vi "Process.vi"(11 "Actor":refnum<class "Main View.lvclass">) -> ()   [LabVIEW 2021, in "Main View.lvclass"]
uses:
  Main View.lvclass
  Element/Element.lvclass/Element.ctl
  Motion/Motion.lvclass/Motion.ctl
  Vector 2D/Vector 2D.lvclass/Vector 2D.ctl
  Re-use Libraries/Minimal Actor Framework/Actors/Base Actor/Actor/Front Panel State.ctl
  Re-use Libraries/Minimal Actor Framework/Actors/Base Actor/Actor/Actor.lvclass
  Re-use Libraries/Minimal Actor Framework/Messaging/Message/Message.lvclass
  Actors/Error Handler/API/Error Handler Actor API.lvclass
  Re-use Libraries/Utility/Utility.lvlib
  Actors/Main Controller/API/Main Controller Actor API.lvclass
  Actors/Main Controller/Actor/Player.ctl
  Actors/Main Controller/Actor/Main Controller Actor.lvclass
  Globals.vi
  Element/Element.lvclass
  Motion/Motion.lvclass
  Vector 2D/Vector 2D.lvclass
  Actors/Main Controller/Actor/Player Icon.ctl
panel:
  in  "Player 2 Position":cluster{"X":i32, "Y":i32}={"X"=2000, "Y"=2000} {"Y" scale=0.0..6400.0; "X" scale=0.0..8192.0}
  in  "Player 1 Position":cluster{"X":i32, "Y":i32}={"X"=1000, "Y"=1000} {"Y" scale=0.0..6400.0; "X" scale=0.0..8192.0}
  in  "Player 2":T1=1
  in  "Player 1":T1
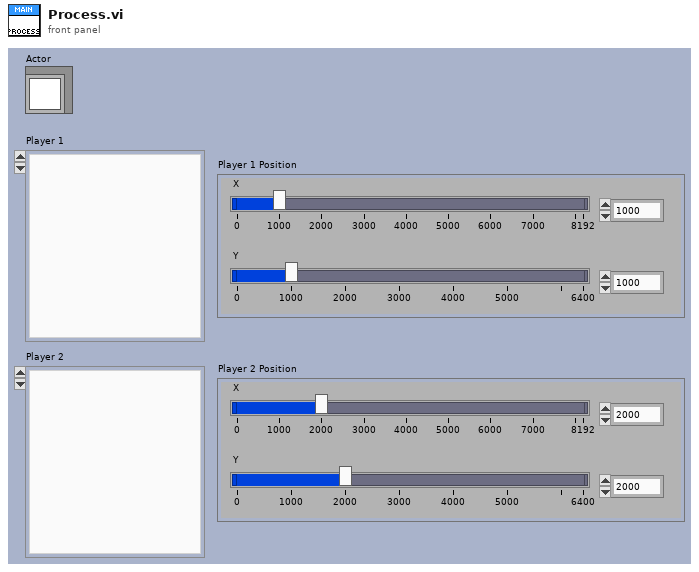
[diagram p1: front panel]
types:
  T1 = typedef "Main Controller Actor.lvclass/Player Icon.ctl" = u16
  T2 = typedef "Actor.lvclass/Front Panel State.ctl" = enum32{"Invalid", "Standard", "Closed", "Hidden", "Minimized", "Maximized"}
  T3 = typedef "Main Controller Actor.lvclass/Player.ctl" = enum16{"1", "2"}
  T4 = cluster{"Actor":refnum<event-registration>, "Main Controller":refnum<event-registration>}
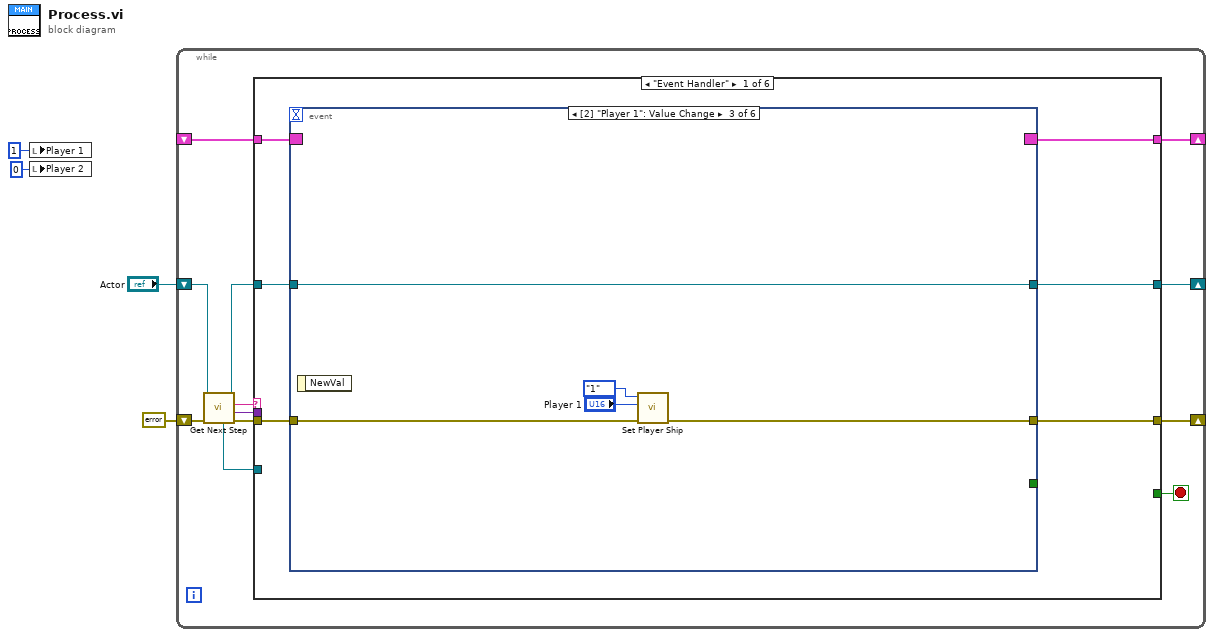
[diagram p0: block diagram]
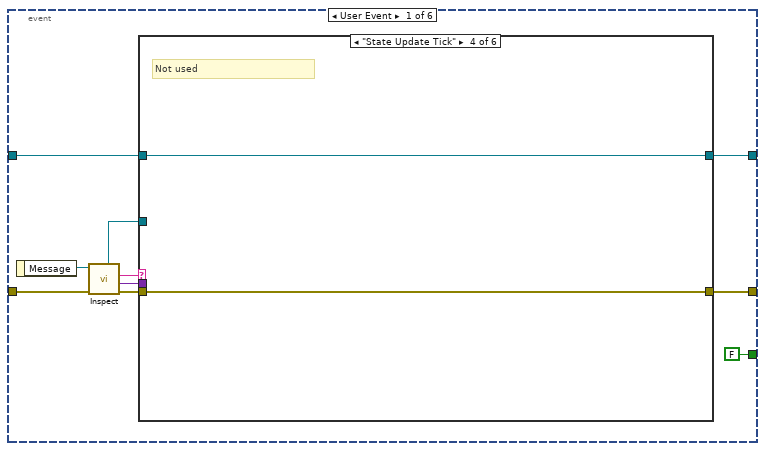
[diagram p2: hidden frame]
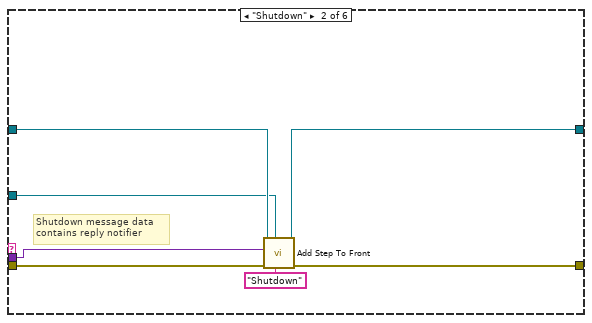
[diagram p4: hidden frame]
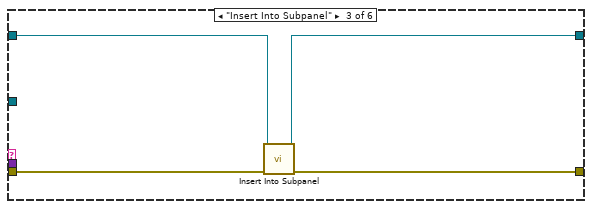
[diagram p5: hidden frame]
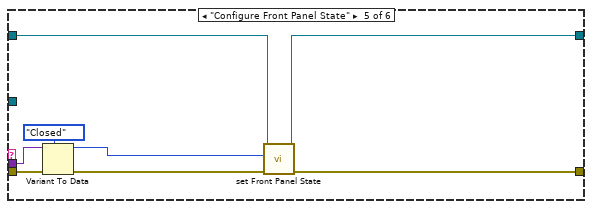
[diagram p6: hidden frame]
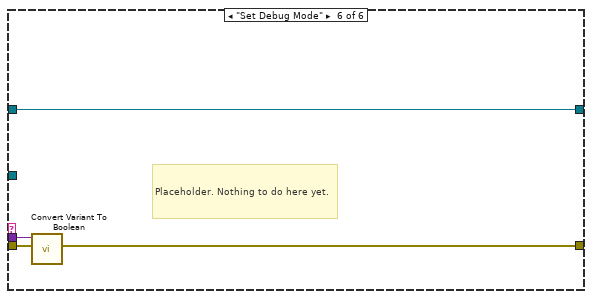
[diagram p7: hidden frame]
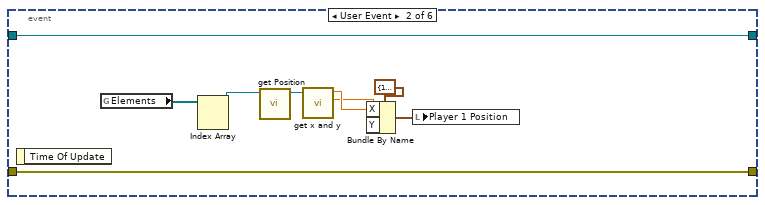
[diagram p8: hidden frame]
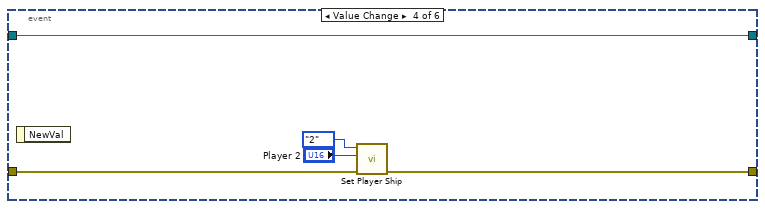
[diagram p9: hidden frame]
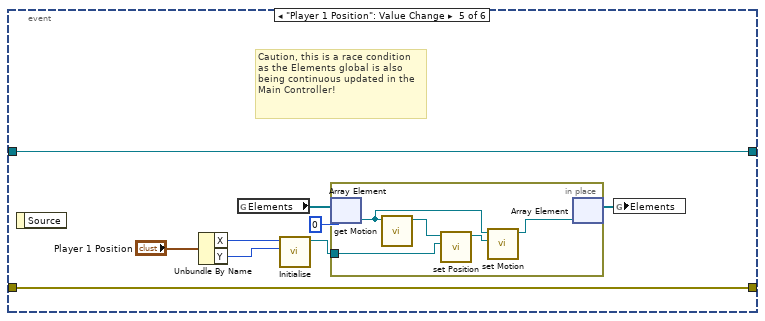
[diagram p10: hidden frame]
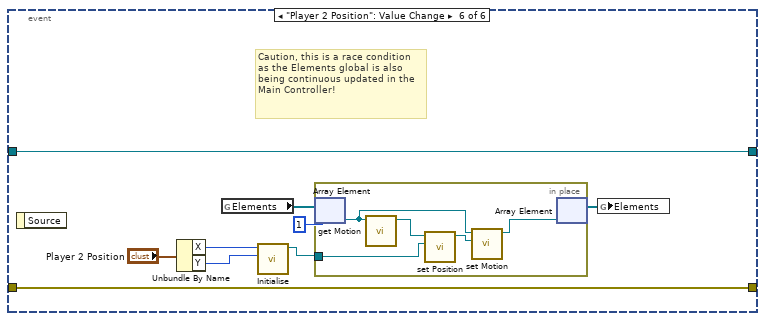
[diagram p11: hidden frame]
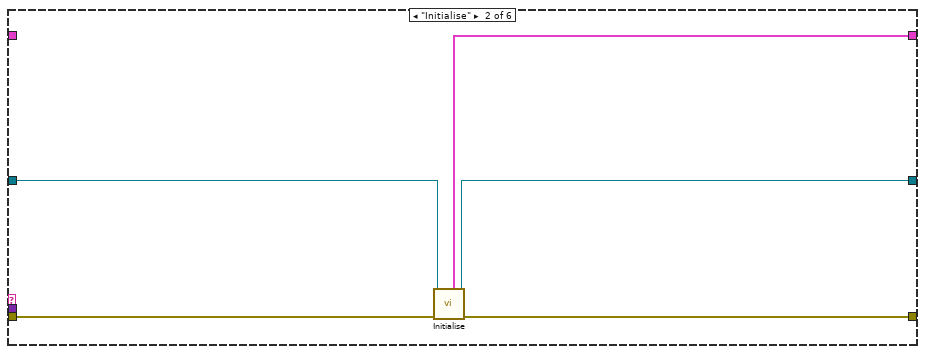
[diagram p12: hidden frame]
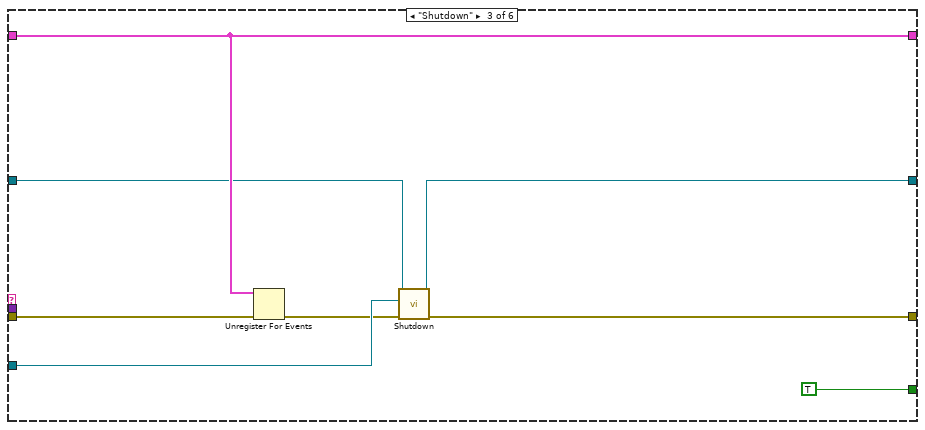
[diagram p13: hidden frame]
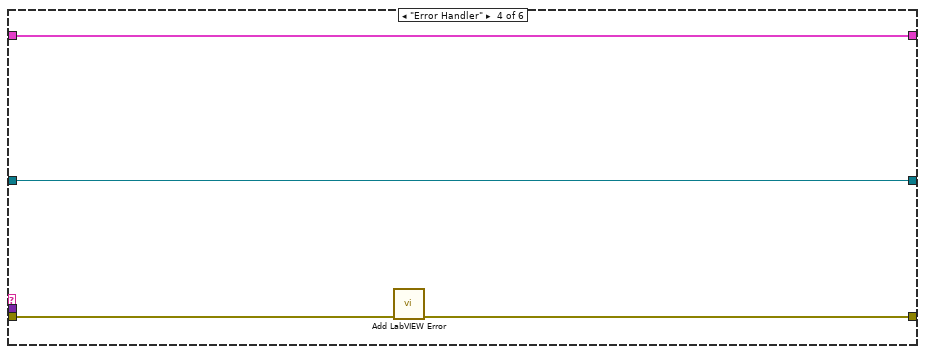
[diagram p14: hidden frame]
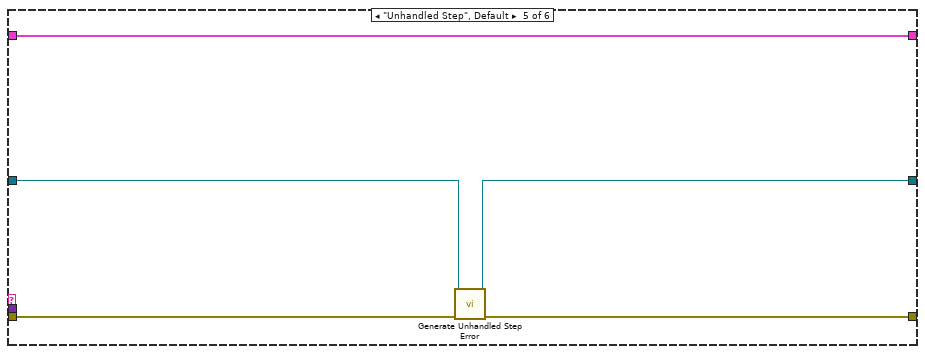
[diagram p15: hidden frame]
diagram:
  n1 = local write "Player 1"(T1 1 ("Player 1")) -> ()
  n2 = local write "Player 2"(T1 0 ("Player 2")) -> ()
  n3 = while {
    shift-right: [w7] -> _
    shift-left: "Actor" -> [w15]
    shift-right: [w12] -> _
    shift-left: _ -> [w11]
    shift-right: [w6] -> _
    shift-left: errorcluster {"status"=FALSE, "code"=0, "source"=""} ("error constant") -> [w9]
    stop <- w16 stop-if-true
    n4 = call-dynamic "Get Next Step.vi"("error in (no error)"=w9, "Actor in"=w15) -> ("error out"=w10:errorcluster, "Parameter"=w13:variant, "Step"=w8:string, "Actor out"=w14:refnum<class "Main View.lvclass">, "Reply Channel"=w5:refnum<notifier>)  [unwired: 5 in]
    n5 = case shown="\"Event Handler\"" w8 {
      tunnel: [_ _ TRUE _ _ _] -> w16
      tunnel: w14 -> [w22 w109 w117 w120 w127 w130]
      tunnel: [w21 w108 w116 w120 w126 w130] -> w7
      tunnel: w13 -> [_ _ _ _ _ _]
      tunnel: [w19 w111 w118 w123 w128 w131] -> w12
      tunnel: w11 -> [w20 _ w118 w123 w128 w131]
      tunnel: w10 -> [w18 w110 w114 w122 w125 w129]
      tunnel: [w17 w107 w112 w121 w124 w129] -> w6
      tunnel: w5 -> [_ _ w115 _ _ _]
      frame "Event Handler" {
        n6 = event shown="[2] \"Player 1\": Value Change" {
          selector: w20 -> [_ _ _ _ _ _]
          dyn-events: [_ _ _ _ _ _] -> w19
          timeout: _ -> [_ _ _ _ _ _]
          tunnel: w22 -> [w32 w68 w73 w78 w83 w101]
          tunnel: [w31 w68 w73 w78 w83 w101] -> w21
          tunnel: w18 -> [w29 w67 w71 w76 w87 w100]
          tunnel: [w30 w67 w70 w75 w87 w100] -> w17
          tunnel: [FALSE _ _ _ _ _] -> _
          event User Event {
            n7 = event-data() -> ("Message"=w28:refnum<class "Message.lvclass">)  [unwired: 1 in]
            n8 = call "Inspect.vi"("error in (no error)"=w29, "Message in"=w28) -> ("error out"=w25:errorcluster, "Data"=w26:variant, "Name"=w27:string, "Reply Channel"=w24:refnum<notifier>)  [unwired: 5 in, 1 out]
            n9 = case shown="\"State Update Tick\"" w27 {
              tunnel: w32 -> [w34 w41 w45 w47 w55 w59]
              tunnel: [w34 w40 w44 w47 w54 w59] -> w31
              tunnel: w25 -> [w33 w38 w43 w46 w51 w57]
              tunnel: [w33 w37 w42 w46 w53 w56] -> w30
              tunnel: w26 -> [_ w36 _ _ w52 w58]
              tunnel: w24 -> [_ w35 _ _ _ _]
              frame Default {
              }
              frame "Shutdown" {
                # "Shutdown message data contains reply notifier"
                n10 = call-dynamic "Add Step To Front.vi"("Step Name"="Shutdown", "Reply Channel"=w35, "error in (no error)"=w38, "Parameter"=w36, "Actor in"=w41) -> ("error out"=w37:errorcluster, "Actor out"=w40:refnum<class "Main View.lvclass">)  [unwired: 5 in]
              }
              frame "Insert Into Subpanel" {
                n11 = call-dynamic "Insert Into Subpanel.vi"("error in (no error)"=w43, "Actor in"=w45) -> ("error out"=w42:errorcluster, "Actor out"=w44:refnum<class "Main View.lvclass">)  [unwired: 8 in]
              }
              frame "State Update Tick" {
                # "Not used"
              }
              frame "Configure Front Panel State" {
                n12 = Variant To Data(error in=w51, type=Front_Panel_State."Closed" ("Front Panel State"), Variant=w52) -> (data=w48:T2, error out=w50:errorcluster)
                n13 = call-dynamic "set Front Panel State.vi"("error in (no error)"=w50, "Front Panel State"=w48, "Actor in"=w55) -> ("error out"=w53:errorcluster, "Actor out"=w54:refnum<class "Main View.lvclass">)  [unwired: 7 in]
              }
              frame "Set Debug Mode" {
                # "Placeholder. Nothing to do here yet."
                n14 = call "Convert Variant To Boolean.vi"("error in (no error)"=w57, "Variant"=w58) -> ("error out"=w56:errorcluster)  [unwired: 8 in, 1 out]
              }
            }
          }
          event User Event {
            n15 = event-data() -> ()  [unwired: 1 in, 1 out]
            n16 = global read "Globals.vi" "Elements"() -> (w66:refnum<class "Element.lvclass">[])
            n17 = Index Array(array=w66) -> (element #1=w65:refnum<class "Element.lvclass">)  [unwired: 2 in, 1 out]
            n18 = call "get Position.vi"("Element in"=w65) -> ("Position"=w64:refnum<class "Vector 2D.lvclass">)  [unwired: 10 in]
            n19 = call "get x and y.vi"("Vector 2D in"=w64) -> ("y"=w61:sgl, "x"=w62:sgl)  [unwired: 9 in]
            n20 = Bundle By Name(cluster=cluster{"X":i32, "Y":i32} {"X"=1000, "Y"=1000} ("Player 1 Position"), "X"=w62, "Y"=w61) -> (w63:cluster{"X":i32, "Y":i32})
            n21 = local write "Player 1 Position"(w63) -> ()
          }
          event Value Change {
            n22 = event-data() -> ()  [unwired: 1 in, 1 out]
            n23 = call "Set Player Ship.vi"("error in (no error)"=w71, "Ship"="Player 1", "Player"=Player."1") -> ("error out"=w70:errorcluster)  [unwired: 8 in]
          }
          event Value Change {
            n24 = event-data() -> ()  [unwired: 1 in, 1 out]
            n25 = call "Set Player Ship.vi"("error in (no error)"=w76, "Ship"="Player 2", "Player"=Player."2") -> ("error out"=w75:errorcluster)  [unwired: 8 in]
          }
          event "Player 1 Position": Value Change {
            # "Caution, this is a race condition as the Elements global is also being continuous updated in the Main Controller!"
            n26 = event-data() -> ()  [unwired: 1 in, 1 out]
            n27 = Unbundle By Name("Player 1 Position") -> ("X"=w81:i32, "Y"=w80:i32)
            n28 = global read "Globals.vi" "Elements"() -> (w86:refnum<class "Element.lvclass">[])
            n29 = call "Initialise.vi"("y"=w80, "x"=w81) -> ("Vector 2D out"=w79:refnum<class "Vector 2D.lvclass">)  [unwired: 9 in]
            n30 = in-place {
              in-place-border: w79 -> [w89]
              n31 = in-place-array #1(w86, 0) -> (w90:refnum<class "Element.lvclass">)
              n32 = call "get Motion.vi"("Element in"=w90) -> ("Motion"=w92:refnum<class "Motion.lvclass">)  [unwired: 10 in]
              n33 = call "set Position.vi"("Position"=w89, "Motion in"=w92) -> ("Motion out"=w91:refnum<class "Motion.lvclass">)  [unwired: 9 in]
              n34 = call "set Motion.vi"("Motion"=w91, "Element in"=w90) -> ("Element out"=w88:refnum<class "Element.lvclass">)  [unwired: 9 in]
              n35 = in-place-array #1(w88) -> (w85:refnum<class "Element.lvclass">[])  [unwired: 1 out]
            }
            n36 = global write "Globals.vi" "Elements"(w85) -> ()
          }
          event "Player 2 Position": Value Change {
            # "Caution, this is a race condition as the Elements global is also being continuous updated in the Main Controller!"
            n37 = event-data() -> ()  [unwired: 1 in, 1 out]
            n38 = Unbundle By Name("Player 2 Position") -> ("X"=w96:i32, "Y"=w95:i32)
            n39 = global read "Globals.vi" "Elements"() -> (w99:refnum<class "Element.lvclass">[])
            n40 = call "Initialise.vi"("y"=w95, "x"=w96) -> ("Vector 2D out"=w93:refnum<class "Vector 2D.lvclass">)  [unwired: 9 in]
            n41 = in-place {
              in-place-border: w93 -> [w103]
              n42 = in-place-array #2(w99, 1) -> (w104:refnum<class "Element.lvclass">)
              n43 = call "get Motion.vi"("Element in"=w104) -> ("Motion"=w106:refnum<class "Motion.lvclass">)  [unwired: 10 in]
              n44 = call "set Position.vi"("Position"=w103, "Motion in"=w106) -> ("Motion out"=w105:refnum<class "Motion.lvclass">)  [unwired: 9 in]
              n45 = call "set Motion.vi"("Motion"=w105, "Element in"=w104) -> ("Element out"=w102:refnum<class "Element.lvclass">)  [unwired: 9 in]
              n46 = in-place-array #2(w102) -> (w98:refnum<class "Element.lvclass">[])  [unwired: 1 out]
            }
            n47 = global write "Globals.vi" "Elements"(w98) -> ()
          }
        }
      }
      frame "Initialise" {
        n48 = call "Initialise.vi"("error in (no error)"=w110, "Actor in"=w109) -> ("error out"=w107:errorcluster, "Actor out"=w108:refnum<class "Main View.lvclass">, "Observers"=w111:T4)  [unwired: 7 in]
      }
      frame "Shutdown" {
        n49 = Unregister For Events(event registration refnum=w118, error in=w114) -> (error out=w113:errorcluster)
        n50 = call-dynamic "Shutdown.vi"("error in (no error)"=w113, "Reply Channel"=w115, "Actor in"=w117) -> ("error out"=w112:errorcluster, "Actor out"=w116:refnum<class "Main View.lvclass">)  [unwired: 7 in]
      }
      frame "Error Handler" {
        n51 = call "Add LabVIEW Error.vi"("error in (no error)"=w122) -> ("error out"=w121:errorcluster)  [unwired: 10 in]
      }
      frame "Unhandled Step", Default {
        n52 = call-dynamic "Generate Unhandled Step Error.vi"("error in (no error)"=w125, "Actor in"=w127) -> ("error out"=w124:errorcluster, "Actor out"=w126:refnum<class "Main View.lvclass">)  [unwired: 8 in]
      }
      frame "-----------------------" {
        # "Separator"
      }
    }
  }
